vi "Scripting_FollowWireDownStreams.vi"(0 "Term Refnum":refnum<vi>, 2 "NodeTypesToFind":string[](array[string]), 3 "CreateParentTerminals(False)":bool, 5 "error in":errorcluster, 6 "MainitainDataType":bool, 7 "StopCriteria":T1) -> (15 "Nodes":refnum<vi>[](array[refnum]), 16 "NodeTypes":string[](array[string]), 17 "ParentTerminal":refnum<vi>[](array[refnum]), 19 "error out":errorcluster)   [LabVIEW 2020]
uses:
  <resource>/Framework/Providers/Open_GDS/ClassProviders/Common/ScriptingFunctions/Scripting_FollowWireDownStreams_StopCriteria.ctl
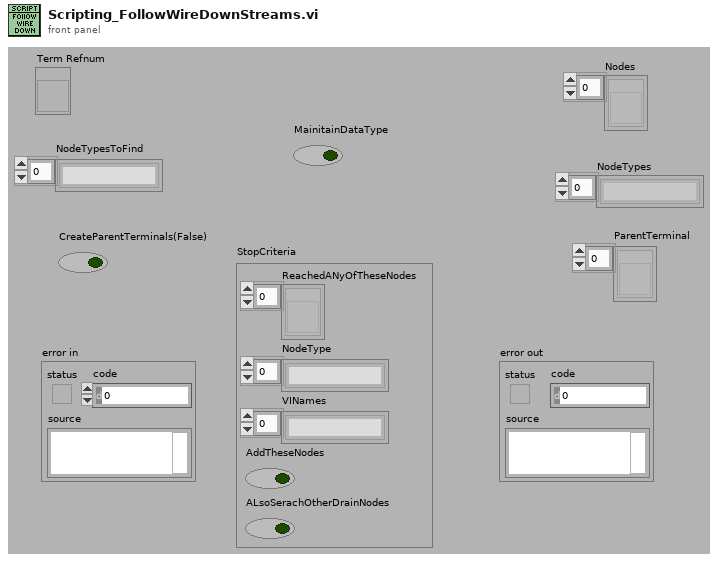
[diagram p1: front panel]
types:
  T1 = typedef "Scripting_FollowWireDownStreams_StopCriteria.ctl" = cluster{"ReachedANyOfTheseNodes":refnum<vi>[], "NodeType":string[], "VINames":string[], "AddTheseNodes":bool, "ALsoSerachOtherDrainNodes":bool}
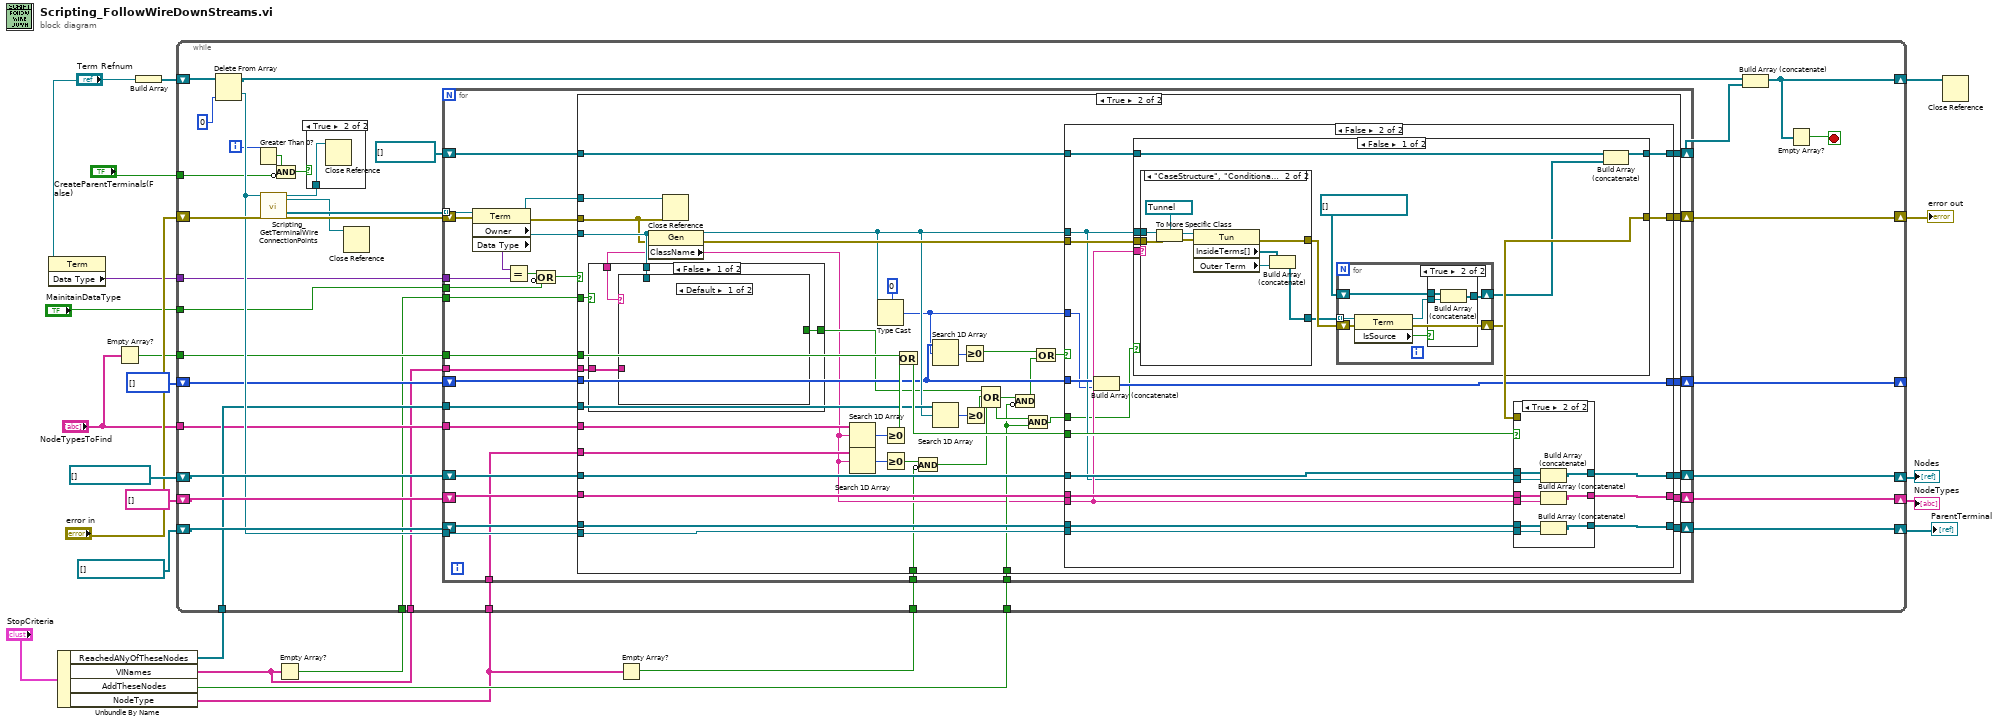
[diagram p0: block diagram]
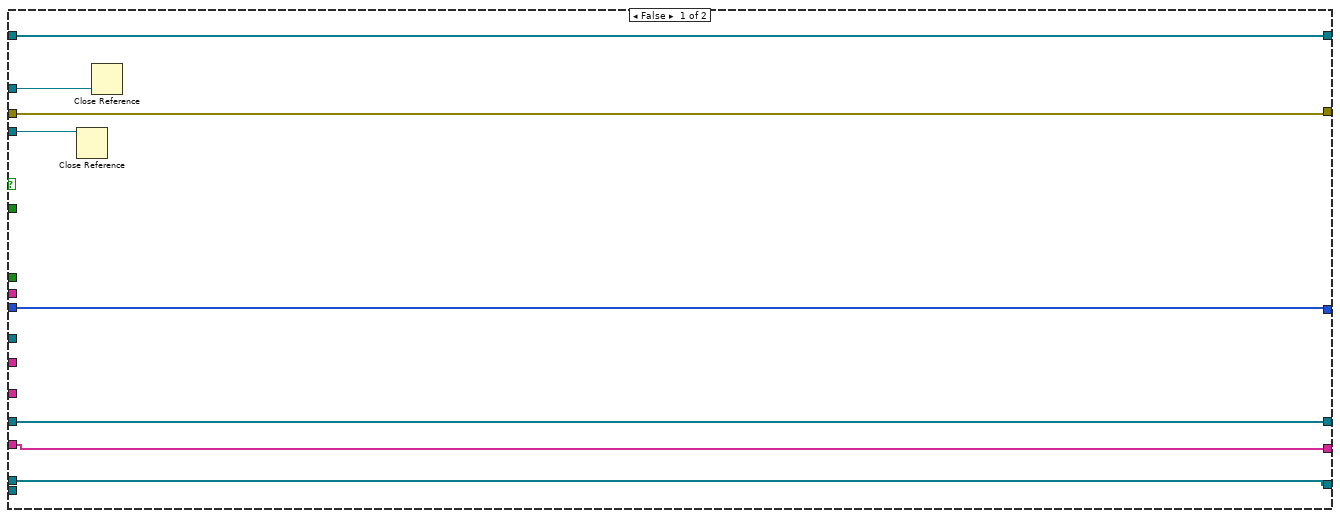
[diagram p3: hidden frame]
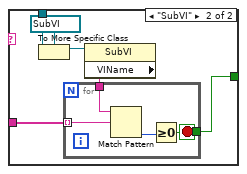
[diagram p4: hidden frame]
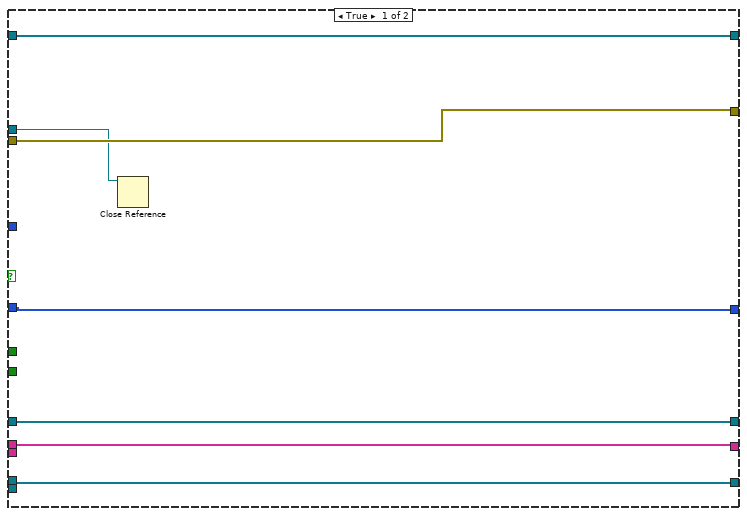
[diagram p6: hidden frame]
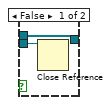
[diagram p7: hidden frame]
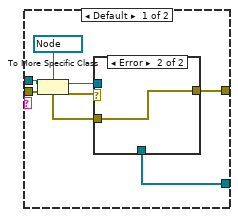
[diagram p8: hidden frame]
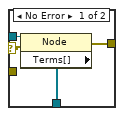
[diagram p9: hidden frame]
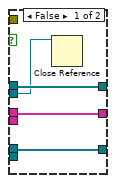
[diagram p11: hidden frame]
diagram:
  n1 = property class="Term"(reference="Term Refnum") -> ("Data Type"=w1:variant)  [unwired: 1 in, 2 out]
  n2 = Unbundle By Name("StopCriteria") -> ("ReachedANyOfTheseNodes"=w12:refnum<vi>[], "VINames"=w7:string[], "AddTheseNodes"=w6:bool, "NodeType"=w5:string[])
  n3 = Empty Array?(array="NodeTypesToFind") -> (empty?=w9:bool)
  n4 = Build Array("Term Refnum") -> (w23:refnum<vi>[])
  n5 = Empty Array?(array=w7) -> (empty?=w8:bool)
  n6 = Empty Array?(array=w5) -> (empty?=w4:bool)
  n7 = while {
    shift-right: [w50] -> w24
    shift-left: w23 -> [w60]
    tunnel: "NodeTypesToFind" -> [w36]
    shift-right: [w53] -> w19
    shift-left: refnum<vi>[] [] -> [w54]
    shift-right: [w52] -> w21
    shift-left: "error in" -> [w51]
    shift-right: [w46] -> w17
    shift-left: string[] [] -> [w45]
    shift-right: [w43] -> w16
    shift-left: refnum<vi>[] [] ("ParentTerminal") -> [w44]
    tunnel: "CreateParentTerminals(False)" -> [w39]
    tunnel: w12 -> [w37]
    shift-right: [w34] -> _
    shift-left: u32[] [] -> [w35]
    tunnel: w9 -> [w32]
    tunnel: w8 -> [w31]
    tunnel: w7 -> [w30]
    tunnel: w6 -> [w29]
    tunnel: w5 -> [w28]
    tunnel: w4 -> [w27]
    tunnel: "MainitainDataType" -> [w26]
    tunnel: w1 -> [w25]
    i -> [w41]
    stop <- w49 stop-if-true
    n8 = Delete From Array(array=w60, index=0) -> (deleted portion=w42:refnum<vi>, array with subset deleted=w59:refnum<vi>[])  [unwired: 1 in]
    n9 = Greater Than 0?(x=w41) -> (x > 0?=w40:bool)
    n10 = call <resource>:"Scripting_GetTerminalWireConnectionPoints.vi"("Term Refnum In"=w42, "error in"=w51) -> ("Term Refnum Out"=w48:refnum<vi>, "WireTermSource"=w47:refnum<vi>, "AllWireTerminalDrains"=w57:refnum<vi>[], "error out"=w56:errorcluster)  [unwired: 9 in, 5 out]
    n11 = Compound Arithmetic op=AND(w40, invert w39) -> (w38:bool)
    n12 = case shown="True" w38 {
      tunnel: w48 -> [_ w61]
      frame False {
      }
      frame True {
        n13 = Close Reference(reference=w61) -> ()  [unwired: 1 in, 1 out]
      }
    }
    n14 = Close Reference(reference=w47) -> ()  [unwired: 1 in, 1 out]
    n15 = for {
      tunnel: w57 -> [w91] mode=indexing
      tunnel: w36 -> [w79]
      shift-right: [w89] -> w53
      shift-left: w54 -> [w90]
      shift-right: [w83] -> w52
      shift-left: w56 -> [w88]
      shift-right: [w87] -> w55
      shift-left: refnum<vi>[] [] -> [w86]
      shift-right: [w85] -> w46
      shift-left: w45 -> [w84]
      shift-right: [w81] -> w43
      shift-left: w44 -> [w82]
      tunnel: w42 -> [w80]
      tunnel: w37 -> [w77]
      tunnel: w32 -> [w78]
      shift-right: [w76] -> w34
      shift-left: w35 -> [w75]
      tunnel: w31 -> [w74]
      tunnel: w30 -> [w72]
      tunnel: w29 -> [w71]
      tunnel: w28 -> [w68]
      tunnel: w27 -> [w67]
      tunnel: w25 -> [w65]
      tunnel: w26 -> [w63]
      n16 = property class="Term"(reference=w91, error in=w88) -> (reference out=w69:refnum<vi>, error out=w70:errorcluster, "Owner"=w73:refnum<vi>, "Data Type"=w66:variant)
      n17 = Equal?(x=w66, y=w65) -> (x = y?=w64:bool)
      n18 = Compound Arithmetic op=OR(w64, invert w63) -> (w62:bool)
      n19 = case shown="True" w62 {
        tunnel: w90 -> [w97 w142]
        tunnel: [w97 w141] -> w89
        tunnel: [w92 w140] -> w87
        tunnel: w86 -> [w92 w139]
        tunnel: [w96 w137] -> w85
        tunnel: w84 -> [w96 w136]
        tunnel: [w93 w134] -> w83
        tunnel: w82 -> [w95 w133]
        tunnel: [w95 w132] -> w81
        tunnel: w80 -> [_ w131]
        tunnel: w79 -> [_ w130]
        tunnel: w78 -> [_ w129]
        tunnel: w77 -> [_ w126]
        tunnel: [w94 w125] -> w76
        tunnel: w75 -> [w94 w122]
        tunnel: w74 -> [_ w116]
        tunnel: w73 -> [w98 w115]
        tunnel: w72 -> [_ w114]
        tunnel: w71 -> [_ w109]
        tunnel: w70 -> [w93 w107]
        tunnel: w69 -> [w99 w106]
        tunnel: w68 -> [_ w104]
        tunnel: w67 -> [_ w101]
        frame False {
          n20 = Close Reference(reference=w98) -> ()  [unwired: 1 in, 1 out]
          n21 = Close Reference(reference=w99) -> ()  [unwired: 1 in, 1 out]
        }
        frame True {
          n22 = property class="Gen"(reference=w115, error in=w107) -> (reference out=w124:refnum<vi>, error out=w135:errorcluster, "ClassName"=w103:string)
          n23 = case shown="False" w116 {
            tunnel: w103 -> [w146 _]
            tunnel: w115 -> [w145 _]
            tunnel: w114 -> [w144 _]
            tunnel: [w143 _] -> w112
            frame False {
              n24 = case shown="Default" w146 {
                tunnel: w145 -> [_ w152]
                tunnel: w144 -> [_ w148]
                tunnel: [_ w147] -> w143
                frame Default {
                }
                frame "SubVI" {
                  n25 = To More Specific Class(target class=refnum<vi> refnum ("Owner"), reference=w152) -> (specific class reference=w150:refnum<vi>)  [unwired: 1 in, 1 out]
                  n26 = property class="SubVI"(reference=w150) -> ("VIName"=w149:string)  [unwired: 1 in, 2 out]
                  n27 = for {
                    tunnel: w149 -> [w156]
                    tunnel: w148 -> [w155] mode=indexing
                    tunnel: [w153] -> w147
                    stop <- w153 stop-if-true
                    n28 = Match Pattern(string=w156, regular expression=w155) -> (offset past match=w154:i32)  [unwired: 1 in, 3 out]
                    n29 = Greater Or Equal To 0?(x=w154) -> (x >= 0?=w153:bool)
                  }
                }
              }
            }
            frame True {
            }
          }
          n30 = Close Reference(reference=w106, error in (no error)=w107) -> ()  [unwired: 1 out]
          n31 = Search 1D Array(1D array=w130, element=w103) -> (index of element=w138:i32)  [unwired: 1 in]
          n32 = Search 1D Array(1D array=w104, element=w103) -> (index of element=w105:i32)  [unwired: 1 in]
          n33 = Type Cast(type=u32 0 ("index"), x=w124) -> (*(type *) &x=w121:u32)
          n34 = Greater Or Equal To 0?(x=w138) -> (x >= 0?=w128:bool)
          n35 = Greater Or Equal To 0?(x=w105) -> (x >= 0?=w102:bool)
          n36 = Or(x=w129, y=w128) -> (x .or. y?=w127:bool)
          n37 = Compound Arithmetic op=AND(w102, invert w101) -> (w100:bool)
          n38 = Search 1D Array(1D array=w122, element=w121) -> (index of element=w119:i32)  [unwired: 1 in]
          n39 = Search 1D Array(1D array=w126, element=w124) -> (index of element=w120:i32)  [unwired: 1 in]
          n40 = Greater Or Equal To 0?(x=w119) -> (x >= 0?=w118:bool)
          n41 = Greater Or Equal To 0?(x=w120) -> (x >= 0?=w113:bool)
          n42 = Compound Arithmetic op=OR(w112, w113, w100) -> (w110:bool)
          n43 = Compound Arithmetic op=AND(w110, invert w109) -> (w111:bool)
          n44 = Compound Arithmetic op=AND(w110, w109) -> (w108:bool)
          n45 = Compound Arithmetic op=OR(w118, w111) -> (w117:bool)
          n46 = case shown="False" w117 {
            tunnel: w142 -> [w161 w181]
            tunnel: [w161 w180] -> w141
            tunnel: [w163 w179] -> w140
            tunnel: w139 -> [w163 w178]
            tunnel: w127 -> [_ w177]
            tunnel: [w160 w176] -> w137
            tunnel: w136 -> [w160 w175]
            tunnel: w135 -> [w162 w174]
            tunnel: w103 -> [_ w173]
            tunnel: [w162 w169] -> w134
            tunnel: w133 -> [w159 w172]
            tunnel: [w159 w171] -> w132
            tunnel: w131 -> [_ w170]
            tunnel: w124 -> [w158 w167]
            tunnel: w122 -> [w157 w168]
            tunnel: [w157 w166] -> w125
            tunnel: w121 -> [_ w165]
            tunnel: w108 -> [_ w164]
            frame True {
              n47 = Close Reference(reference=w158) -> ()  [unwired: 1 in, 1 out]
            }
            frame False {
              n48 = Build Array (concatenate)(w168, w165) -> (w166:u32[])
              n49 = case shown="False" w164 {
                tunnel: [w191 w225] -> w179
                tunnel: w178 -> [w190 w225]
                tunnel: w174 -> [w189 w226]
                tunnel: w173 -> [w188 _]
                tunnel: [w185 w226] -> w169
                tunnel: w167 -> [w183 _]
                frame False {
                  n50 = case shown="\"CaseStructure\", \"ConditionalTunnel\", \"LeftShiftRegister\", \"LoopTunnel\", \"RightShiftRegister\", \"SelectorTunnel\", \"Tunnel\"" w188 {
                    tunnel: w189 -> [w204 w223]
                    tunnel: [w207 w220] -> w187
                    tunnel: w183 -> [w208 w219]
                    tunnel: [w206 w216] -> w186
                    frame Default {
                      n51 = To More Specific Class(target class=refnum<vi> refnum ("Owner"), reference=w208, error in=w204) -> (specific class reference=w209:refnum<vi>, error out=w205:errorcluster)
                      n52 = case shown="Error" w205 {
                        selector: w205 -> [w211 _]
                        tunnel: w209 -> [w214 _]
                        tunnel: [w213 w215] -> w207
                        tunnel: [w212 _] -> w206
                        tunnel: w204 -> [_ w215]
                        frame No Error {
                          n53 = property class="Node"(reference=w214, error in=w211) -> (error out=w213:errorcluster, "Terms[]"=w212:refnum<vi>[])  [unwired: 1 out]
                        }
                        frame Error {
                        }
                      }
                    }
                    frame "CaseStructure", "ConditionalTunnel", "LeftShiftRegister", "LoopTunnel", "RightShiftRegister", "SelectorTunnel", "Tunnel" {
                      n54 = To More Specific Class(target class=refnum<vi> refnum ("reference"), reference=w219, error in=w223) -> (specific class reference=w222:refnum<vi>, error out=w221:errorcluster)
                      n55 = property class="Tun"(reference=w222, error in=w221) -> (error out=w220:errorcluster, "InsideTerms[]"=w218:refnum<vi>[], "Outer Term"=w217:refnum<vi>)  [unwired: 1 out]
                      n56 = Build Array (concatenate)(w218, w217) -> (w216:refnum<vi>[])
                    }
                  }
                  n57 = for {
                    tunnel: w186 -> [w198] mode=indexing
                    shift-right: [w196] -> w185
                    shift-left: w187 -> [w197]
                    shift-right: [w192] -> w184
                    shift-left: refnum<vi>[] [] -> [w195]
                    n58 = property class="Term"(reference=w198, error in=w197) -> (reference out=w193:refnum<vi>, error out=w196:errorcluster, "IsSource"=w194:bool)
                    n59 = case shown="True" w194 {
                      tunnel: w195 -> [w200 w203]
                      tunnel: w193 -> [w199 w202]
                      tunnel: [w200 w201] -> w192
                      frame False {
                        n60 = Close Reference(reference=w199) -> ()  [unwired: 1 in, 1 out]
                      }
                      frame True {
                        n61 = Build Array (concatenate)(w203, w202) -> (w201:refnum<vi>[])
                      }
                    }
                  }
                  n62 = Build Array (concatenate)(w190, w184) -> (w191:refnum<vi>[])
                }
                frame True {
                }
              }
              n63 = case shown="True" w177 {
                tunnel: w181 -> [w230 w239]
                tunnel: [w230 w238] -> w180
                tunnel: w173 -> [_ w235]
                tunnel: w175 -> [w229 w236]
                tunnel: [w229 w237] -> w176
                tunnel: w167 -> [w228 w234]
                tunnel: w169 -> [_ _]
                tunnel: w170 -> [_ w233]
                tunnel: w172 -> [w227 w232]
                tunnel: [w227 w231] -> w171
                frame False {
                  n64 = Close Reference(reference=w228) -> ()  [unwired: 1 in, 1 out]
                }
                frame True {
                  n65 = Build Array (concatenate)(w239, w234) -> (w238:refnum<vi>[])
                  n66 = Build Array (concatenate)(w236, w235) -> (w237:string[])
                  n67 = Build Array (concatenate)(w232, w233) -> (w231:refnum<vi>[])
                }
              }
            }
          }
        }
      }
    }
    n68 = Build Array (concatenate)(w59, w55) -> (w50:refnum<vi>[])
    n69 = Empty Array?(array=w50) -> (empty?=w49:bool)
  }
  "error out" <- w21
  "Nodes" <- w19
  "NodeTypes" <- w17
  "ParentTerminal" <- w16
  n70 = Close Reference(reference=w24) -> ()  [unwired: 1 in, 1 out]
